vi "Parse Recursive From XML.vi"(7 "Parent Path (empty)":string, 10 "XML String":string, 11 "Tree Map In":T1) -> (0 "Path Invalid":bool, 2 "XML String Out":string, 3 "Tree Map Out":T1)   [LabVIEW 2021, in "Tree Map.lvlib"]
doc: "<b>Author:</b> Piotr Kruczkowski <PrimaryKey>\n<b>License:</b> NewBSD\n\nCopyright (c) 2019, National Instruments\nAll rights reserved.\n\nRedistribution and use in source and binary forms, with or without\nmodification, are permitted provided that the following conditions are met:\n1. Redistributions of source code must retain the above copyright\n notice, this list of conditions and the following disclaimer.\n2. Redistributions in binary form must reproduce the above copyright\n notice, this list of conditions and the following disclaimer in the\n documentation and/or other materials provided with the distribution.\n3. Neither the name of National Instruments nor the\n names of its contributors may be used to endorse or promote products\n derived from this software without specific prior written permission.\n\nTHIS SOFTWARE IS PROVIDED BY National Instruments ''AS IS'' AND ANY\nEXPRESS OR IMPLIED WARRANTIES, INCLUDING, BUT NOT LIMITED TO, THE IMPLIED\nWARRANTIES OF MERCHANTABILITY AND FITNESS FOR A PARTICULAR PURPOSE ARE\nDISCLAIMED. IN NO EVENT SHALL National Instruments BE LIABLE FOR ANY\nDIRECT, INDIRECT, INCIDENTAL, SPECIAL, EXEMPLARY, OR CONSEQUENTIAL DAMAGES\n(INCLUDING, BUT NOT LIMITED TO, PROCUREMENT OF SUBSTITUTE GOODS OR SERVICES;\nLOSS OF USE, DATA, OR PROFITS; OR BUSINESS INTERRUPTION) HOWEVER CAUSED AND\nON ANY THEORY OF LIABILITY, WHETHER IN CONTRACT, STRICT LIABILITY, OR TORT\n(INCLUDING NEGLIGENCE OR OTHERWISE) ARISING IN ANY WAY OUT OF THE USE OF THIS\nSOFTWARE, EVEN IF ADVISED OF THE POSSIBILITY OF SUCH DAMAGE."
uses:
  <vilib>/National Instruments/Tree Map/Tree Map.lvlib
  <vilib>/National Instruments/Tree Map/Tree Map Data.ctl
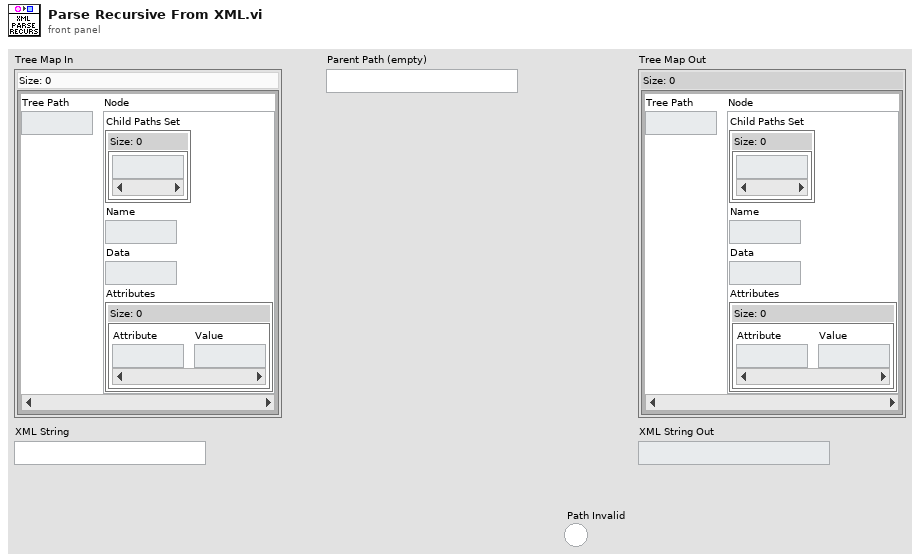
[diagram p1: front panel]
types:
  T1 = typedef "Tree Map.lvlib/Tree Map Data.ctl" = map{string, cluster{"Child Paths Set":set{string}, "Name":string, "Data":string, "Attributes":map{string, string}}}
  T2 = cluster{"Nothing?":bool, "Ignore?":bool, "Closing Tag?":bool, "Finished Tag?":bool, "No Matching Bracket?":bool}
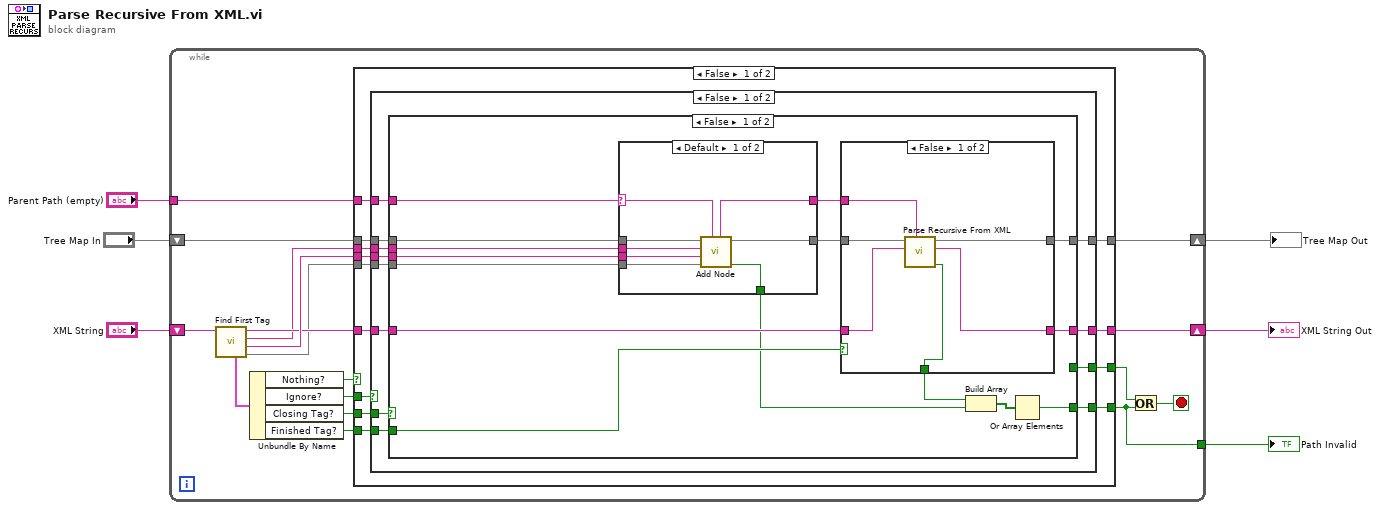
[diagram p0: block diagram]
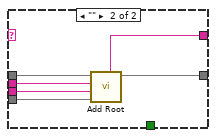
[diagram p3: hidden frame]
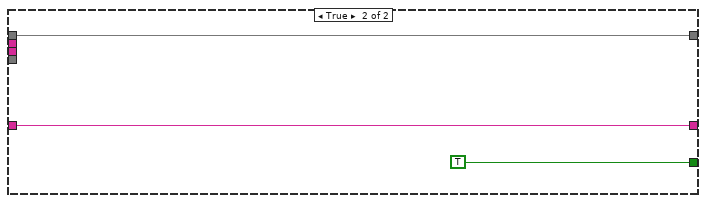
[diagram p4: hidden frame]
diagram:
  n1 = while {
    shift-right: [w12] -> w6
    shift-left: "XML String" -> [w23]
    tunnel: "Parent Path (empty)" -> [w16]
    shift-right: [w19] -> w1
    shift-left: "Tree Map In" -> [w20]
    tunnel: [w10] -> w3
    stop <- w11 stop-if-true
    n2 = call <vilib>:"Find First Tag.vi"("XML String"=w23) -> ("Attributes"=w7:map{string, string}, "Data"=w15:string, "Tag Name"=w8:string, "XML After First Tag"=w13:string, "Flags"=w21:T2)  [unwired: 6 in]
    n3 = Unbundle By Name(w21) -> ("Nothing?"=w22:bool, "Ignore?"=w18:bool, "Closing Tag?"=w17:bool, "Finished Tag?"=w14:bool)
    n4 = case shown="False" w22 {
      selector: w22 -> [_ w91]
      tunnel: [w36 w93] -> w19
      tunnel: w20 -> [w35 w93]
      tunnel: w18 -> [w34 _]
      tunnel: w17 -> [w33 _]
      tunnel: w16 -> [w32 _]
      tunnel: w8 -> [w31 _]
      tunnel: w15 -> [w30 _]
      tunnel: w14 -> [w29 _]
      tunnel: w13 -> [w28 w92]
      tunnel: [w27 w92] -> w12
      tunnel: [w26 _] -> w10
      tunnel: [w25 w91] -> w9
      tunnel: w7 -> [w24 _]
      frame False {
        n5 = case shown="False" w34 {
          tunnel: [w47 w90] -> w36
          tunnel: w35 -> [w46 w90]
          tunnel: w33 -> [w48 _]
          tunnel: w32 -> [w45 _]
          tunnel: w31 -> [w44 _]
          tunnel: w30 -> [w43 _]
          tunnel: w29 -> [w42 _]
          tunnel: w28 -> [w41 w89]
          tunnel: [w40 w89] -> w27
          tunnel: [w39 _] -> w26
          tunnel: [w38 _] -> w25
          tunnel: w24 -> [w37 _]
          frame False {
            n6 = case shown="False" w48 {
              tunnel: [w57 w88] -> w47
              tunnel: w46 -> [w62 w88]
              tunnel: w45 -> [w63 _]
              tunnel: w44 -> [w61 _]
              tunnel: w43 -> [w60 _]
              tunnel: w42 -> [w59 _]
              tunnel: w41 -> [w56 w87]
              tunnel: [w55 w87] -> w40
              tunnel: [w51 _] -> w39
              tunnel: [_ TRUE] -> w38
              tunnel: w37 -> [w49 _]
              frame False {
                n7 = case shown="Default" w63 {
                  selector: w63 -> [w77 _]
                  tunnel: w62 -> [w79 w85]
                  tunnel: w61 -> [w76 w80]
                  tunnel: w60 -> [w75 w81]
                  tunnel: [w78 w84] -> w58
                  tunnel: [w73 w83] -> w54
                  tunnel: [w72 _] -> w52
                  tunnel: w49 -> [w74 w82]
                  frame Default {
                    n8 = call <vilib>:"Add Node.vi"("Parent Path"=w77, "Attributes"=w74, "Data"=w75, "New Node Name"=w76, "Tree Map In"=w79) -> ("Path Invalid"=w72:bool, "Tree Map Out"=w78:T1, "New Node Path"=w73:string)  [unwired: 4 in]
                  }
                  frame "" {
                    n9 = call <vilib>:"Add Root.vi"("Root Attributes"=w82, "Root Data"=w81, "New Root Name"=w80, "Tree Map In"=w85) -> ("Tree Map Out"=w84:T1, "Root Path"=w83:string)  [unwired: 6 in]
                  }
                }
                n10 = case shown="False" w59 {
                  tunnel: w58 -> [w65 w71]
                  tunnel: [w69 w71] -> w57
                  tunnel: w56 -> [w68 w70]
                  tunnel: [w67 w70] -> w55
                  tunnel: w54 -> [w66 _]
                  tunnel: [w64 _] -> w50
                  frame False {
                    n11 = call <vilib>:"Parse Recursive From XML.vi"("Parent Path (empty)"=w66, "XML String"=w68, "Tree Map In"=w65) -> ("Path Invalid"=w64:bool, "XML String Out"=w67:string, "Tree Map Out"=w69:T1)  [unwired: 6 in]
                  }
                  frame True {
                  }
                }
                n12 = Build Array(w50, w52) -> (w53:bool[])
                n13 = Or Array Elements(Boolean array=w53) -> (logical OR=w51:bool)
              }
              frame True {
              }
            }
          }
          frame True {
          }
        }
      }
      frame True {
      }
    }
    n14 = Or(x=w9, y=w10) -> (x .or. y?=w11:bool)
  }
  "XML String Out" <- w6
  "Path Invalid" <- w3
  "Tree Map Out" <- w1
